vi "Test_feed_forward1.vi"() -> ()   [LabVIEW 2013]
uses:
  Input_5782/5782_Fast_PID_states.ctl
  <vilib>/Platform/TimedLoop/XDataNode/timing_clust.ctl
  <vilib>/Platform/TimedLoop/XDataNode/nitl_modes.ctl
  <vilib>/Platform/TimedLoop/XDataNode/wakeup.ctl
  <vilib>/rvi/Emulation/niFpgaSctlEmulationGetInTimedLoop.vi
  <vilib>/rvi/Emulation/niFpgaEmulationReportErrorSimple.vi
  <vilib>/rvi/Emulation/niFpgaGetClockAttributes.vi
  <vilib>/rvi/eio/common/nirviEmuTemplateMethod_errors.vi
  <vilib>/rvi/Emulation/niFpgaCriticalErrorInLSC.vi
  <vilib>/rvi/interface/RandomDataEmulation/nirviRandomDataFPGAFIFO.vi
  <vilib>/rvi/interface/RandomDataEmulation/niFpgaRandomDataHandleErrors.vi
  <vilib>/Platform/TimedLoop/XDataNode/XDataNode.xnode
  <vilib>/eio/EIONode/EIONode.xnode
  <vilib>/rvi/DataTransferAndStorage/Container/XNode/niFpgaContainer.xnode
  <vilib>/rvi/interface/RandomDataEmulation/nirviRandomDataFpgaReadWriteTemplate.vi
  <vilib>/Platform/TimedLoop/XDataNode/XDNodeRunTimeDep.lvlib
panel:
  out "IO Module\\Trigger Input":bool
  in  "Beam enabled":bool
  in  "Trigger Acquisition":bool
  in  "IO Module\\AO Data Sync":bool=TRUE
  in  "IO Module\\SPI Write Data":u16
  out "IO Module\\SPI Read Data":u8
  in  "IO Module\\SPI Read":bool
  in  "IO Module\\SPI Write":bool
  in  "IO Module\\SPI Address":u16
  in  "IO Module\\SPI Device":u8
  out "IO Module\\SPI Idle":bool
  in  "User Command Commit":bool
  in  "User Command":u8
  out "User Command Idle":bool
  out "User Command Status":u8
  in  "User Data 0":u8
  in  "User Data 1":u8
  out "PLL Locked":bool
  out "User Error":bool
  out "Configured?":bool
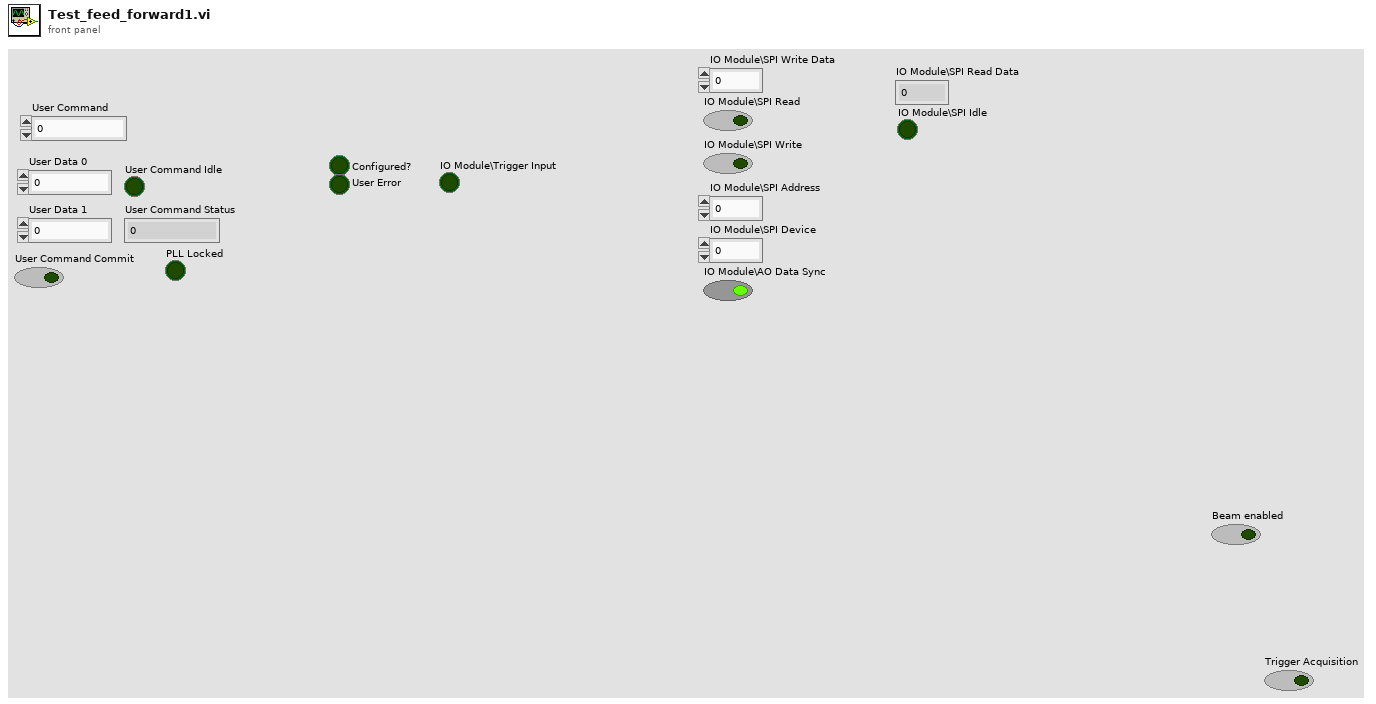
[diagram p1: front panel]
types:
  T1 = typedef "5782_Fast_PID_states.ctl" = enum8{"Wait for trigger", "Acquisition", "Send record length", "Wait for output", "Quiet period"}
  T2 = typedef "XDNodeRunTimeDep.lvlib/timing_clust.ctl" = cluster{"Expected End [f-1]":u64, "Actual End [f-1]":u64, "Finished Late? [f-1]":bool, "Expected End [i-1]":u64, "Actual End [i-1]":u64, "Finished Late? [i-1]":bool, "Expected Start [i]":u64, "Actual Start [i]":u64, "Expected Start [f]":u64, "Actual Start [f]":u64, "Source Name":string, "Structure Name":string, "Period":i64, "Deadline":i64, "Offset":i64, "Start":i64, "Priority":i32, "Timeout":i32, "Mode":T3, "Wakeup Reason":T4, "Error":errorcluster, "Source Type":string, "Secondary Source Type":string, "Global End Time":u64, "Global Start Time":u64, "Frame Duration":u64, "Iteration Duration":u64, "Assigned CPU":i32, "I/O Scan Engine Mode":u32}
  T3 = typedef "XDNodeRunTimeDep.lvlib/nitl_modes.ctl" = enum32{"No Change", "Process missed periods, maintain original phase", "Discard missed periods, maintain original phase", "Process missed periods, ignore original phase", "Discard missed periods, ignore original phase"}
  T4 = typedef "XDNodeRunTimeDep.lvlib/wakeup.ctl" = enum32{"Normal", "Aborted", "Asynchronous wakeup", "Timing source error", "Timed loop error", "Timeout"}
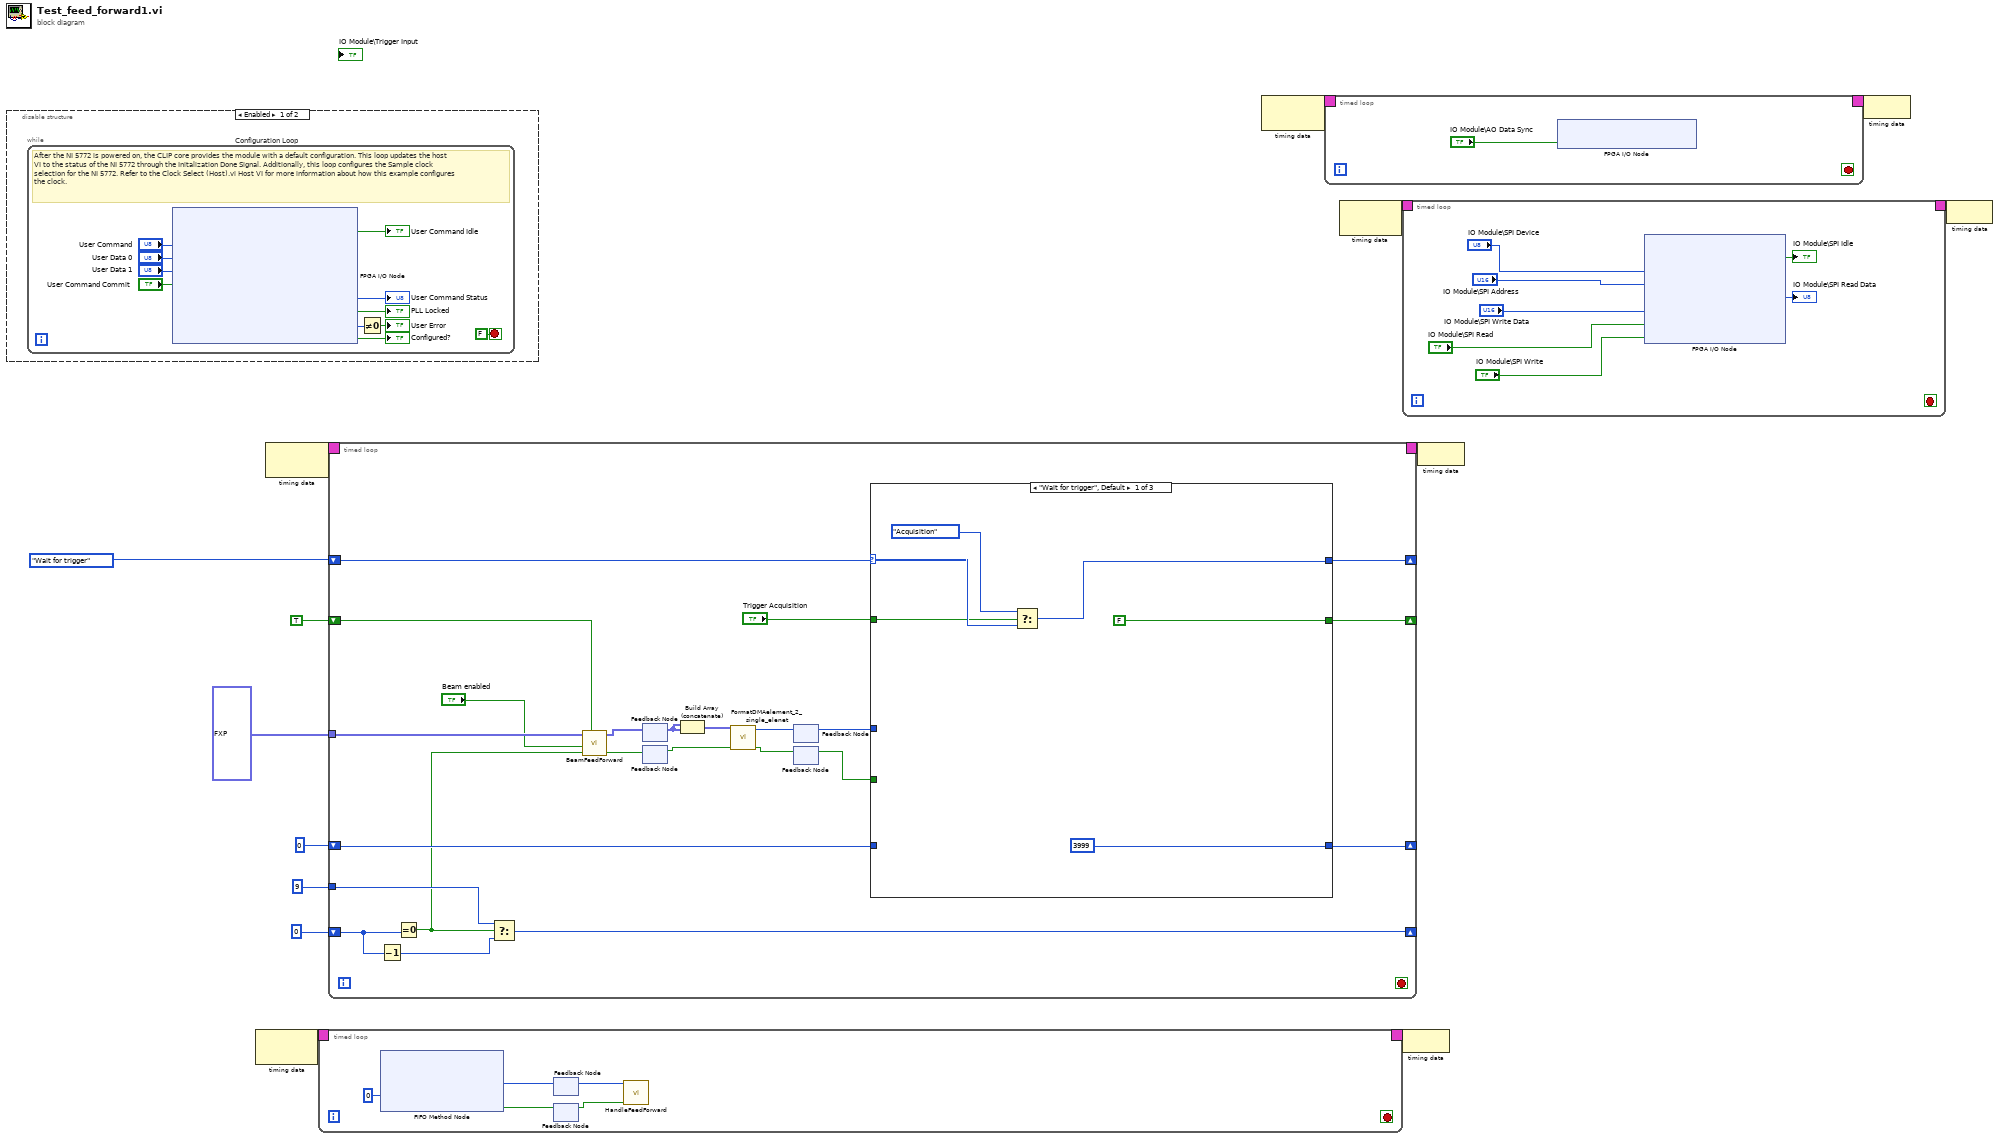
[diagram p0: block diagram]
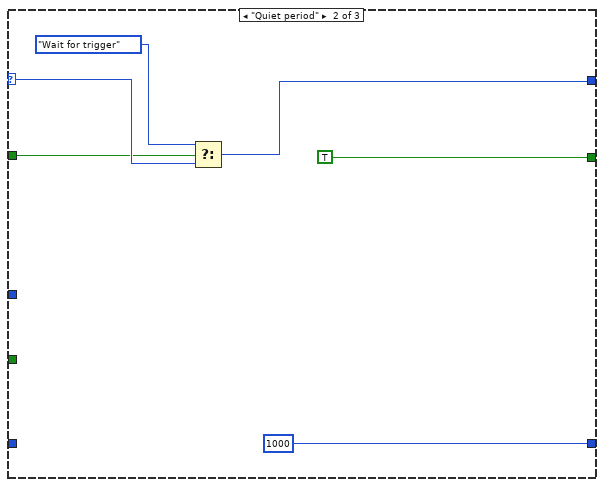
[diagram p2: hidden frame]
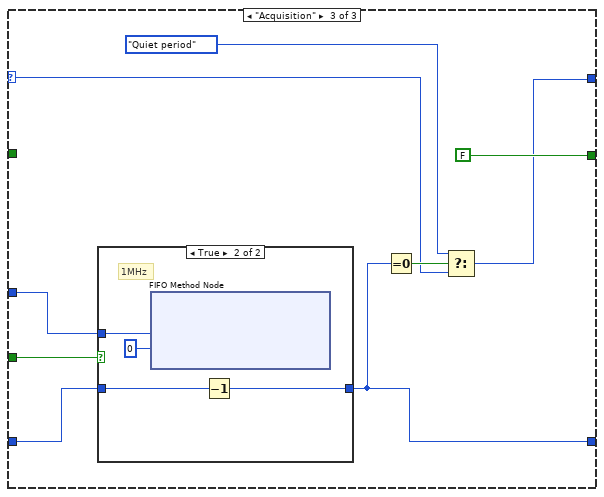
[diagram p3: hidden frame]
diagram:
  n1 = disable-structure shown="Enabled" {
    frame Enabled {
      n2 = while "Configuration Loop" {
        stop <- FALSE stop-if-true
        # "After the NI 5772 is powered on, the CLIP core provides the module with a default configuration. This loop updates the host VI to the status of the NI 5772 through the Initalization Done Signal. Additionally, this loop configures the Sample clock selection for the NI 5772. Refer to the Clock Select (Host).vi Host VI for more information about how this example configures the clock."
        n3 = xnode "FPGA I/O Node"("IO Module\\User Command"="User Command", "IO Module\\User Data 0"="User Data 0", "IO Module\\User Data 1"="User Data 1", "IO Module\\User Command Commit"="User Command Commit") -> ("IO Module\\User Command Idle"=→"User Command Idle":bool, "IO Module\\User Command Status"=→"User Command Status":u8, "IO Module\\PLL Locked"=→"PLL Locked":bool, "IO Module\\User Error"=w20:u8, "IO Module\\Initialization Done"=→"Configured?":bool)  [unwired: 9 in, 9 out]
        n4 = Not Equal To 0?(x=w20) -> (x != 0?=→"User Error":bool)
      }
    }
    frame Disabled {
    }
  }
  n5 = node-c288() -> (w14:T2)  [unwired: 1 in]
  n6 = node-c288() -> (w8:T2)  [unwired: 1 in]
  n7 = timed-loop {
    timing: w14 -> [_]
    timing-out: [_] -> w13
    stop <- _ stop-if-true
    n8 = xnode ("FIFO Method Node")("Timeout"=0) -> ("Element"=w29:u64, "Timed Out?"=w27:bool)  [unwired: 1 in, 1 out]
    n9 = feedback #1() -> (w28:u64)  [unwired: 1 in]
    n10 = feedback-in #1(w29) -> ()
    n11 = feedback #2() -> (w26:bool)  [unwired: 1 in]
    n12 = feedback-in #2(w27) -> ()
    n13 = call "HandleFeedForward.vi"("timed out"=w26, "Value"=w28) -> ()  [unwired: 10 in]
  }
  n14 = timed-loop {
    timing: w8 -> [_]
    timing-out: [_] -> w7
    shift-right: [w48] -> _
    shift-left: TRUE -> [w45]
    shift-right: [w52] -> _
    shift-left: u16 0 -> [w54]
    tunnel: u16 9 -> [w55]
    shift-right: [w49] -> _
    shift-left: 5782_Fast_PID_states."Wait for trigger" ("5782 states") -> [w51]
    shift-right: [w50] -> _
    shift-left: u32 0 -> [w46]
    tunnel: fxp<+/-,16,14>[] [1.0, 1.0] ("Data in") -> [w43]
    stop <- _ stop-if-true
    n15 = Decrement(x=w54) -> (x-1=w53:u16)
    n16 = Equal To 0?(x=w54) -> (x = 0?=w44:bool)
    n17 = Select(t=w55, s=w44, f=w53) -> (s? t:f=w52:u16)
    n18 = call "BeamFeedForward.vi"("Reset"=w45, "input valid"=w44, "beam enabled"="Beam enabled", "Data in"=w43) -> ("output valid"=w40:bool, "Data out"=w41:fxp<+/-,16,14>[])  [unwired: 6 in]
    n19 = feedback #3() -> (w39:fxp<+/-,16,14>[])  [unwired: 1 in]
    n20 = feedback-in #3(w41) -> ()
    n21 = feedback #4() -> (w38:bool)  [unwired: 1 in]
    n22 = feedback-in #4(w40) -> ()
    n23 = Build Array (concatenate)(w39, w39) -> (w37:fxp<+/-,16,14>[])
    n24 = call "FormatDMAelement_2_single_elenet.vi"("valid in"=w38, "Data in"=w37) -> ("valid out"=w34:bool, "Element"=w36:u64)  [unwired: 8 in]
    n25 = feedback #5() -> (w35:u64)  [unwired: 1 in]
    n26 = feedback-in #5(w36) -> ()
    n27 = feedback #6() -> (w33:bool)  [unwired: 1 in]
    n28 = feedback-in #6(w34) -> ()
    n29 = case shown="\"Wait for trigger\", Default" w51 {
      selector: w51 -> [w59 w65 w70]
      tunnel: w46 -> [_ _ w76]
      tunnel: [u16 3999 u16 1000 w75] -> w50
      tunnel: [w58 w64 w68] -> w49
      tunnel: [FALSE TRUE FALSE] -> w48
      tunnel: w33 -> [_ _ w74]
      tunnel: w35 -> [_ _ w73]
      tunnel: "Trigger Acquisition" -> [w56 w62 _]
      frame "Wait for trigger", Default {
        n30 = Select(t=5782_Fast_PID_states."Acquisition" ("5782 states"), s=w56, f=w59) -> (s? t:f=w58:T1)
      }
      frame "Quiet period" {
        n31 = Select(t=5782_Fast_PID_states."Wait for trigger" ("5782 states"), s=w62, f=w65) -> (s? t:f=w64:T1)
      }
      frame "Acquisition" {
        n32 = case shown="True" w74 {
          tunnel: w73 -> [_ w81]
          tunnel: [w77 w78] -> w75
          tunnel: w76 -> [w77 w79]
          frame False {
          }
          frame True {
            # "1MHz"
            n33 = xnode ("FIFO Method Node")("Element"=w81, "Timeout"=0) -> ()  [unwired: 1 in, 2 out]
            n34 = Decrement(x=w79) -> (x-1=w78:u32)
          }
        }
        n35 = Equal To 0?(x=w75) -> (x = 0?=w71:bool)
        n36 = Select(t=5782_Fast_PID_states."Quiet period", s=w71, f=w70) -> (s? t:f=w68:T1)
      }
    }
  }
  n37 = node-c288() -> (w10:T2)  [unwired: 1 in]
  n38 = timed-loop {
    timing: w10 -> [_]
    timing-out: [_] -> w9
    stop <- _ stop-if-true
    n39 = xnode "FPGA I/O Node"("IO Module\\AO Data Sync"="IO Module\\AO Data Sync") -> ()  [unwired: 1 in, 1 out]
  }
  n40 = node-c288() -> (w12:T2)  [unwired: 1 in]
  n41 = timed-loop {
    timing: w12 -> [_]
    timing-out: [_] -> w11
    stop <- _ stop-if-true
    n42 = xnode "FPGA I/O Node"("IO Module\\SPI Device"="IO Module\\SPI Device", "IO Module\\SPI Address"="IO Module\\SPI Address", "IO Module\\SPI Write Data"="IO Module\\SPI Write Data", "IO Module\\SPI Read"="IO Module\\SPI Read", "IO Module\\SPI Write"="IO Module\\SPI Write") -> ("IO Module\\SPI Idle"=→"IO Module\\SPI Idle":bool, "IO Module\\SPI Read Data"=→"IO Module\\SPI Read Data":u8)  [unwired: 7 in, 7 out]
  }
  n43 = node-c288(w13) -> ()
  n44 = node-c288(w7) -> ()
  n45 = node-c288(w9) -> ()
  n46 = node-c288(w11) -> ()
